vi "Catch Error.vi"(7 "Clear":bool=TRUE, 8 "Error In":errorcluster, 10 "Source":string, 11 "Severity":T1=enum."Recoverable") -> (0 "Error Out":errorcluster)   [LabVIEW 2017, in "Logger.lvlib"]
doc: "Handles an error by converting it to a logging statement and sending to listeners, including the default log file if enabled, based on the configured Level and selected Severity of the error."
uses:
  Logger.lvlib
  Controls/Severity.ctl
  Controls/Tag.ctl
  <vilib>/Utility/error.llb/DialogType.ctl
  Private/Error/Action.ctl
  Private/Action.ctl
  Controls/Statement.ctl
  <vilib>/dlg_ctls.llb/Space Constant.vi
  <vilib>/Utility/error.llb/Trim Whitespace.vi
  Private/Error/Error.lvlib
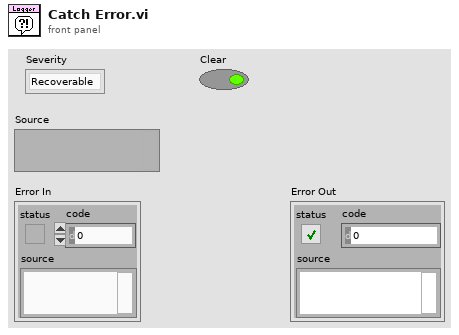
[diagram p1: front panel]
types:
  T1 = typedef "Logger.lvlib/Severity.ctl" = enum16{"Benign", "Warning", "Recoverable", "Fatal"}
  T2 = typedef "Logger.lvlib/Action.ctl" = enum16{"Initialize", "Register", "Log", "Unregister", "Set Level", "Shutdown"}
  T3 = typedef "Logger.lvlib/Error.lvlib/Action.ctl" = enum16{"Initialize", "Get", "Set Verbosity", "Set User-Defined Codes", "Set User-Defined Descriptions", "Shutdown"}
  T4 = typedef "Logger.lvlib/Tag.ctl" = enum16{"Fatal", "Error", "Warn", "Info", "Debug", "Trace"}
  T5 = typedef "Logger.lvlib/Statement.ctl" = cluster{"Time Stamp":timestamp, "Tag":T4, "Source":string, "Message":string}
  T6 = typedef "DialogType.ctl" = u16
  T7 = typedef "Logger.lvlib/Error.lvlib/Data.ctl" = cluster{"Verbosity":u8, "User-Defined Codes":i32[], "User-Defined Descriptions":string[]}
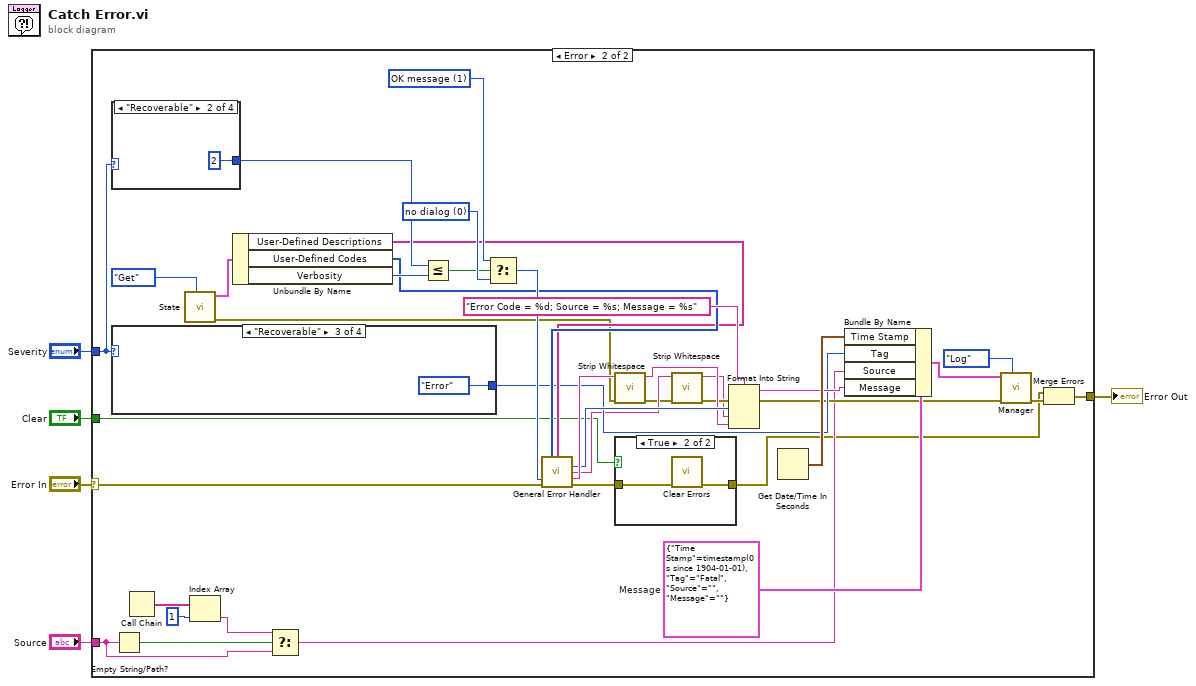
[diagram p0: block diagram]
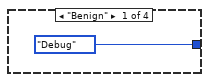
[diagram p4: hidden frame]
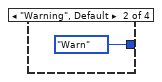
[diagram p5: hidden frame]
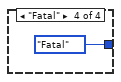
[diagram p6: hidden frame]
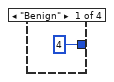
[diagram p7: hidden frame]
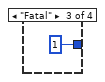
[diagram p8: hidden frame]
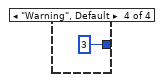
[diagram p9: hidden frame]
diagram:
  n1 = case shown="Error" "Error In" {
    selector: "Error In" -> [w6 w45]
    tunnel: "Severity" -> [_ w37]
    tunnel: [w6 w22] -> w3
    tunnel: "Source" -> [_ w11]
    tunnel: "Clear" -> [_ w7]
    frame No Error {
    }
    frame Error {
      w28 = T5 {"Time Stamp"=timestamp(0 s since 1904-01-01), "Tag"=enum."Fatal", "Source"="", "Message"=""}  # Message
      w44 = T6 0 items=["no dialog", "OK message", "continue or stop message", "OK message + warnings", "continue/stop + warnings"] ("type of dialog (OK msg:1)")
      w43 = T6 1 items=["no dialog", "OK message", "continue or stop message", "OK message + warnings", "continue/stop + warnings"] ("type of dialog (OK msg:1)")
      n2 = case shown="\"Recoverable\"" w37 {
        tunnel: [u8 4 u8 2 u8 1 u8 3] -> w35
        frame "Benign" {
        }
        frame "Recoverable" {
        }
        frame "Fatal" {
        }
        frame "Warning", Default {
        }
      }
      n3 = case shown="\"Recoverable\"" w37 {
        tunnel: [Tag."Debug" ("Level") Tag."Warn" ("Level") Tag."Error" ("Level") Tag."Fatal" ("Level")] -> w24
        frame "Benign" {
        }
        frame "Warning", Default {
        }
        frame "Recoverable" {
        }
        frame "Fatal" {
        }
      }
      n4 = Empty String/Path?(string/path=w11) -> (empty?=w13:bool)
      n5 = Call Chain() -> (call chain=w15:string[])
      n6 = call "State.vi"("Action"=Action."Get") -> ("Error Out"=w30:errorcluster, "Data"=w34:T7)  [unwired: 9 in]
      n7 = Index Array(array=w15, index=1) -> (element=w12:string)
      n8 = Unbundle By Name(w34) -> ("User-Defined Descriptions"=w31:string[], "User-Defined Codes"=w32:i32[], "Verbosity"=w33:u8)
      n9 = Select(t=w12, s=w13, f=w11) -> (s? t:f=w10:string)
      n10 = Less Or Equal?(x=w35, y=w33) -> (x <= y?=w42:bool)
      n11 = Select(t=w43, s=w42, f=w44) -> (s? t:f=w41:T6)
      n12 = call <vilib>:"General Error Handler.vi"("[user-defined codes]"=w32, "[user-defined descriptions]"=w31, "type of dialog (OK msg:1)"=w41, "error in (no error)"=w45) -> ("code out"=w38:i32, "source out"=w23:string, "message"=w39:string, "error out"=w9:errorcluster)  [unwired: 7 in, 1 out]
      n13 = call "Strip Whitespace.vi"("Error In"=w30, "Text"=w39) -> ("Error Out"=w19:errorcluster, "Stripped Text"=w20:string)  [unwired: 8 in]
      n14 = case shown="True" w7 {
        tunnel: w9 -> [w46 w48]
        tunnel: [w46 w47] -> w8
        frame False {
        }
        frame True {
          n15 = call <vilib>:"Clear Errors.vi"("error in (no error)"=w48) -> ("error out"=w47:errorcluster)  [unwired: 5 in, 1 out]
        }
      }
      n16 = call "Strip Whitespace.vi"("Error In"=w19, "Text"=w23) -> ("Error Out"=w18:errorcluster, "Stripped Text"=w16:string)  [unwired: 8 in]
      n17 = Format Into String(format string="Error Code = %d; Source = %s; Message = %s", error in=w18, w38, w16, w20) -> (resulting string=w25:string, error out=w17:errorcluster)  [unwired: 1 in]
      n18 = Get Date/Time In Seconds() -> (seconds since 1Jan1904=w27:timestamp)
      n19 = Bundle By Name(cluster=w28, "Time Stamp"=w27, "Tag"=w24, "Source"=w10, "Message"=w25) -> (w26:T5)
      n20 = call "Manager.vi"("Action"=Action."Log", "Error In"=w17, "Value In"=w26) -> ("Error Out"=w21:errorcluster)  [unwired: 8 in]
      n21 = Merge Errors(w8, w21) -> (w22:errorcluster)
    }
  }
  "Error Out" <- w3
